vi "Create Rubix Cube in 3D Pic Control.vi"(8 "error in (no error)":errorcluster, 10 "Rubix Array":string[][](array[string])) -> (0 "error out":errorcluster, 2 "Rubix Array":refnum<vi>[][](array[refnum]), 3 "Scene:New Object":refnum<vi>)   [LabVIEW 2019]
uses:
  <vilib>/picture/3D Picture Control/Object/Create Object (name).vi
  <vilib>/picture/3D Picture Control/NI_3D Picture Control.lvlib
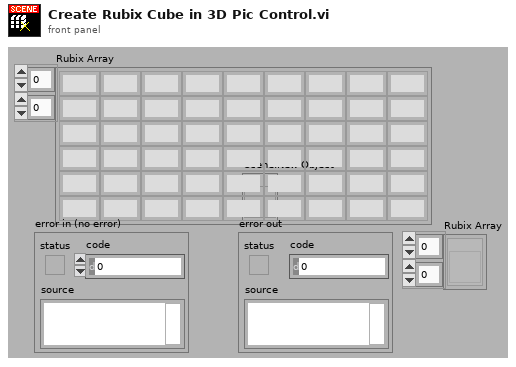
[diagram p1: front panel]
types:
  T1 = cluster{"Axis":cluster{"X":sgl, "Y":sgl, "Z":sgl}, "Angle":sgl}[]
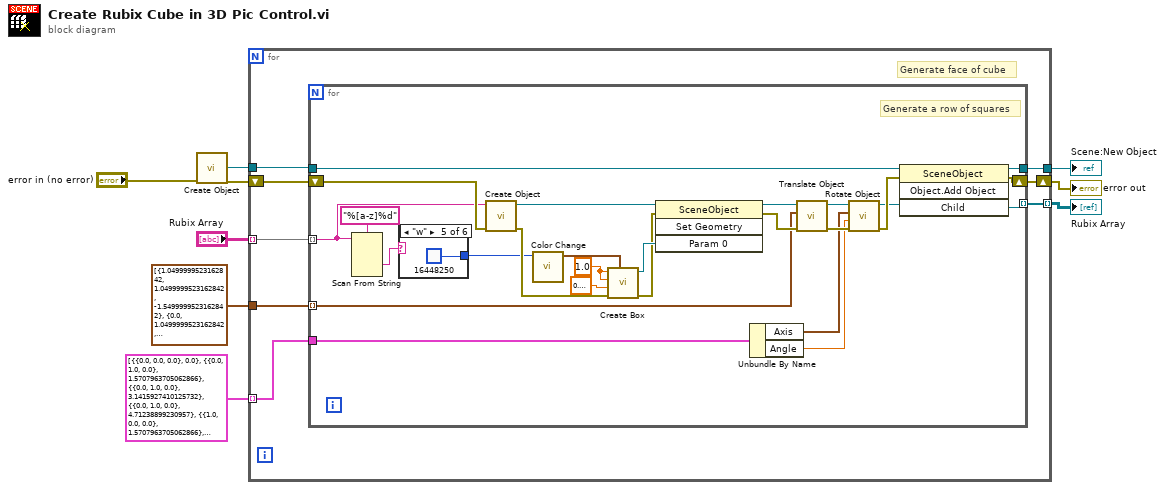
[diagram p0: block diagram]
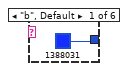
[diagram p2: hidden frame]
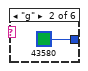
[diagram p3: hidden frame]
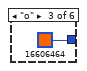
[diagram p4: hidden frame]
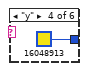
[diagram p5: hidden frame]
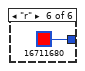
[diagram p6: hidden frame]
diagram:
  n1 = call-poly <vilib>:"Create Object.vi"("error in (no error)"="error in (no error)") -> ("error out"=w6:errorcluster, "Scene:New Object"=w5:refnum<vi>)  [unwired: 9 in]
  n2 = for {
    tunnel: [w17] -> w9
    tunnel: "Rubix Array" -> [w10] mode=indexing
    tunnel: T1 [{"Axis"={"X"=0.0, "Y"=0.0, "Z"=0.0}, "Angle"=0.0}, {"Axis"={"X"=0.0, "Y"=1.0, "Z"=0.0}, "Angle"=1.5707964}, {"Axis"={"X"=0.0, "Y"=1.0, "Z"=0.0}, "Angle"=3.1415927}, {"Axis"={"X"=0.0, "Y"=1.0, "Z"=0.0}, "Angle"=4.712389}, {"Axis"={"X"=1.0, "Y"=0.0, "Z"=0.0}, "Angle"=1.5707964}, {"Axis"={"X"=1.0, "Y"=0.0, "Z"=0.0}, "Angle"=4.712389}] -> [w16] mode=indexing
    tunnel: w5 -> [w15]
    shift-right: [w14] -> w3
    shift-left: w6 -> [w13]
    tunnel: cluster{"X":sgl, "Y":sgl, "Z":sgl}[] [{"X"=1.05, "Y"=1.05, "Z"=-1.55}, {"X"=0.0, "Y"=1.05, "Z"=-1.55}, {"X"=-1.05, "Y"=1.05, "Z"=-1.55}, {"X"=1.05, "Y"=0.0, "Z"=-1.55}, {"X"=0.0, "Y"=0.0, "Z"=-1.55}, {"X"=-1.05, "Y"=0.0, "Z"=-1.55}, {"X"=1.05, "Y"=-1.05, "Z"=-1.55}, {"X"=0.0, "Y"=-1.05, "Z"=-1.55}, {"X"=-1.05, "Y"=-1.05, "Z"=-1.55}] -> [w12]
    tunnel: [w11] -> w1 mode=indexing
    # "Generate face of cube"
    n3 = for {
      tunnel: w12 -> [w26] mode=indexing
      shift-right: [w34] -> w14
      shift-left: w13 -> [w24]
      tunnel: w15 -> [w38]
      tunnel: [w39] -> w17
      tunnel: w10 -> [w19] mode=indexing
      tunnel: w16 -> [w31]
      tunnel: [w20] -> w11 mode=indexing
      w27 = sgl 1.0 ("Length X")
      # "Generate a row of squares"
      n4 = Scan From String(format string="%[a-z]%d", input string=w19) -> (output 1=w21:string)  [unwired: 5 in, 3 out]
      n5 = case shown="\"w\"" w21 {
        tunnel: [u32 1388031 ("Color") u32 43580 ("Color") u32 16606464 ("Color") u32 16048913 ("Color") u32 16448250 ("Color") u32 16711680 ("Color")] -> w23
        frame "b", Default {
        }
        frame "g" {
        }
        frame "o" {
        }
        frame "y" {
        }
        frame "w" {
        }
        frame "r" {
        }
      }
      n6 = call-poly <vilib>:"Create Object.vi"("error in (no error)"=w24, "Name"=w19) -> ("error out"=w37:errorcluster, "Scene:New Object"=w42:refnum<vi>)  [unwired: 8 in]
      n7 = call <vilib>:"Color Change.vi"("Color"=w23) -> ("RGBA"=w43:cluster{"R":sgl, "G":sgl, "B":sgl, "A":sgl})  [unwired: 10 in]
      n8 = call <vilib>:"Create Box.vi"("Color"=w43, "error in (no error)"=w37, "Length Z"=sgl 0.1, "Length Y"=w27, "Length X"=w27) -> ("error out"=w36:errorcluster, "New Box Refnum"=w41:refnum<vi>)  [unwired: 5 in]
      n9 = invoke class="SceneObject" method="Set Geometry"(reference=w42, error in=w36, "Param 0"=w41) -> (reference out=w40:refnum<vi>, error out=w35:errorcluster)  [unwired: 1 in, 2 out]
      n10 = Unbundle By Name(w31) -> ("Axis"=w30:cluster{"X":sgl, "Y":sgl, "Z":sgl}, "Angle"=w29:sgl)
      n11 = call <vilib>:"Translate Object.vi"("error in (no error)"=w35, "Translation"=w26, "Scene.Object In"=w40) -> ("error out"=w32:errorcluster, "Scene.Object Out"=w33:refnum<vi>)  [unwired: 7 in]
      n12 = call <vilib>:"Rotate Object.vi"("error in (no error)"=w32, "Angle"=w29, "Axis"=w30, "Scene.Object In"=w33) -> ("error out"=w25:errorcluster, "Scene.Object Out"=w18:refnum<vi>)  [unwired: 6 in]
      n13 = invoke class="SceneObject" method="Object.Add Object"(reference=w38, error in=w25, "Child"=w18) -> (reference out=w39:refnum<vi>, error out=w34:errorcluster, "Child"=w20:refnum<vi>)  [unwired: 1 in, 1 out]
    }
  }
  "Scene:New Object" <- w9
  "error out" <- w3
  "Rubix Array" <- w1
